vi "Set Config.vi"(8 "error in (no error)":errorcluster, 10 "Reference":refnum<vi>, 11 "DataGrid Config":refnum<class "DataGrid Config.lvclass">) -> (0 "error out":errorcluster, 3 "Tag Set":bool)   [LabVIEW 2018, in "DataGrid Config.lvclass"]
uses:
  DataGrid Config.lvclass
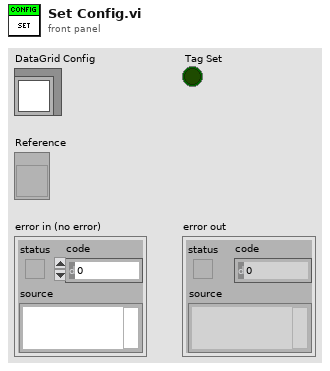
[diagram p1: front panel]
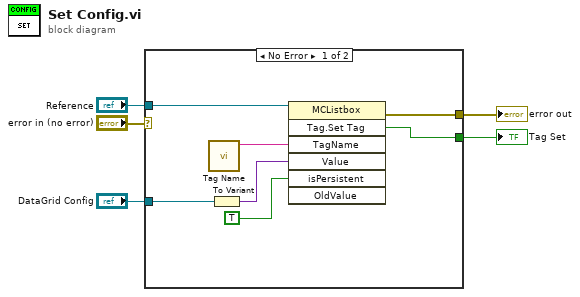
[diagram p0: block diagram]
diagram:
  n1 = case shown="No Error" "error in (no error)" {
    selector: "error in (no error)" -> [_ w13]
    tunnel: [w7 w13] -> w4
    tunnel: [w11 _] -> w3
    tunnel: "DataGrid Config" -> [w10 _]
    tunnel: "Reference" -> [w6 _]
    frame No Error {
      n2 = call "Tag Name.vi"() -> ("String"=w12:string)  [unwired: 11 in]
      n3 = To Variant(anything=w10) -> (Variant=w8:variant)
      n4 = invoke class="MCListbox" method="Tag.Set Tag"(reference=w6, "TagName"=w12, "Value"=w8, "isPersistent"=TRUE) -> (error out=w7:errorcluster, "SetTag"=w11:bool)  [unwired: 3 in, 5 out]
    }
    frame Error {
    }
  }
  "error out" <- w4
  "Tag Set" <- w3
